vi "Update Timestamp.vi"(6 "Offset (-1 default)":i32=-1, 8 "error in (no error)":errorcluster, 9 "New TAI Time (ns)":i64, 10 "Bytes in":u8[](array[numeric]), 11 "pcap Parse and Build in":refnum<class "pcap_Parse_Build_CIF.lvclass">) -> (0 "error out":errorcluster, 2 "Bytes out":u8[](array[numeric]), 3 "pcap Parse and Build out":refnum<class "pcap_Parse_Build_CIF.lvclass">)   [LabVIEW 2021, in "pcap_Parse_Build_CIF.lvclass"]
doc: "Update the timestamp in-line with the byte array. This is useful for changing time offset of existing data. \n\nIf called after the Parse Packet Header then the offset can be left at the default -1. It will automatically back-up one header set from the current offset. If a value other than -1 is provided it will update the bytes at that location. There is no check to verify location in the byte stream so it is possible to corrupt data if incorrect offsets are used."
uses:
  pcap_Parse_Build_CIF.lvclass
  pcap_Parse_Build_CIF.lvclass/pcap_Parse_Build_CIF.ctl
  Typedef/Errors.ctl
  e9022ed4-8435-466f-84f6-b9a136e00ec6.vi
  b7a2a79d-019e-453d-9ead-29c6d68c4f86.vi
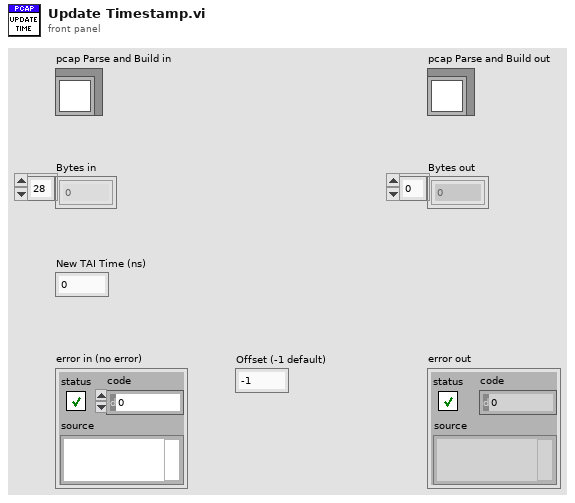
[diagram p1: front panel]
types:
  T1 = typedef "pcap_Parse_Build_CIF.lvclass/Errors.ctl" = enum16{"Invalid Global Header", "Out of Data"}
  T2 = typedef "pcap_Parse_Build_CIF.lvclass/Time Format.ctl" = enum16{"us", "ns"}
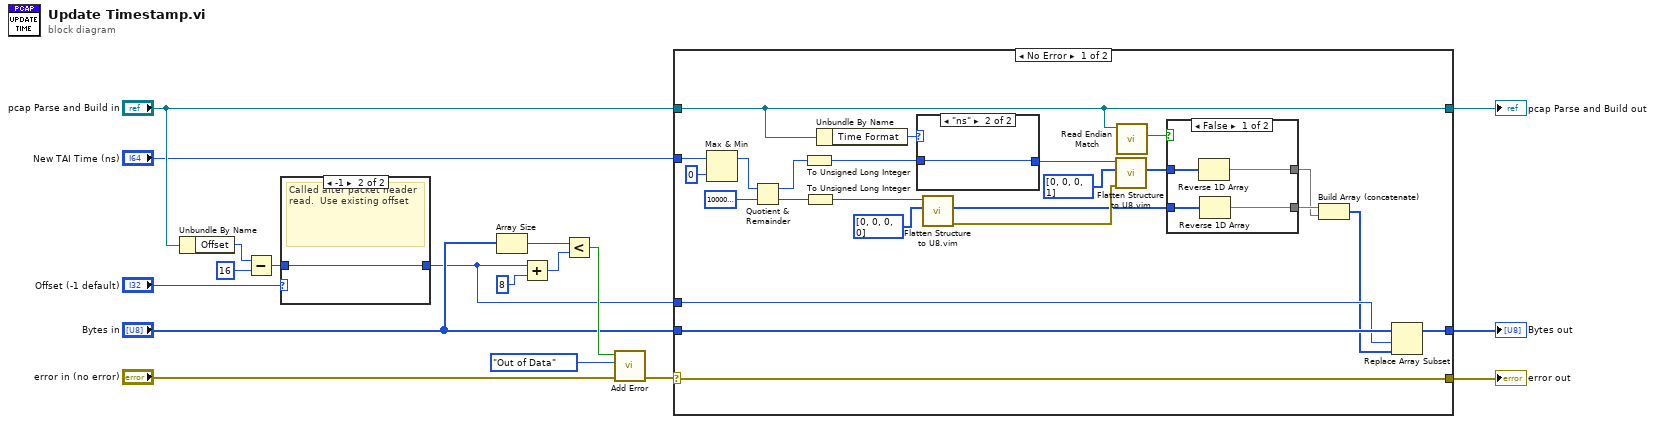
[diagram p0: block diagram]
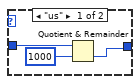
[diagram p4: hidden frame]
diagram:
  n1 = Unbundle By Name("pcap Parse and Build in") -> ("Offset"=w7:i32)
  n2 = Subtract(x=w7, y=16) -> (x-y=w4:i32)
  n3 = case shown="-1" "Offset (-1 default)" {
    selector: "Offset (-1 default)" -> [w18 _]
    tunnel: w4 -> [_ w19]
    tunnel: [w18 w19] -> w3
    frame 0, Default {
      # "Explicit offset provided"
    }
    frame -1 {
      # "Called after packet header read.  Use existing offset"
    }
  }
  n4 = Array Size(array="Bytes in") -> (size(s)=w9:i32)
  n5 = Add(x=w3, y=8 ("length")) -> (x+y=w13:i32)
  n6 = Less?(x=w9, y=w13) -> (x < y?=w11:bool)
  n7 = call "Add Error.vi"("Error"=Errors."Out of Data", "Insert Error"=w11) -> ()  [unwired: 9 in, 1 out]
  n8 = case shown="No Error" "error in (no error)" {
    selector: "error in (no error)" -> [w43 w56]
    tunnel: [w43 w56] -> w16
    tunnel: [w36 w55] -> w14
    tunnel: "pcap Parse and Build in" -> [w36 w55]
    tunnel: "Bytes in" -> [w30 w54]
    tunnel: w3 -> [w29 _]
    tunnel: "New TAI Time (ns)" -> [w37 _]
    tunnel: [w28 w54] -> w1
    frame No Error {
      n9 = Max & Min(x=w37, y=i64 0) -> (max(x,y)=w38:i64)  [unwired: 1 out]
      n10 = Quotient & Remainder(x=w38, y=i64 1000000000) -> (x-y*floor(x/y)=w41:i64, floor(x/y)=w40:i64)
      n11 = To Unsigned Long Integer(number=w41) -> (unsigned 32bit integer=w34:u32)
      n12 = To Unsigned Long Integer(number=w40) -> (unsigned 32bit integer=w33:u32)
      n13 = Unbundle By Name(w36) -> ("Time Format"=w35:T2)
      n14 = case shown="\"ns\"" w35 {
        tunnel: w34 -> [w52 w53]
        tunnel: [w50 w53] -> w31
        frame "us" {
          n15 = Quotient & Remainder(x=w52, y=u32 1000) -> (floor(x/y)=w50:u32)  [unwired: 1 out]
        }
        frame "ns" {
        }
      }
      n16 = call "Flatten Structure to U8.vim"("Flattened Data in"=u8[] [0, 0, 0, 0], "Data to Flatten in"=w33) -> ("error out"=w26:errorcluster, "Flattened Data out"=w22:u8[])  [unwired: 7 in, 1 out]
      n17 = call "Flatten Structure to U8.vim"("error in"=w26, "Flattened Data in"=u8[] [0, 0, 0, 1], "Data to Flatten in"=w31) -> ("Flattened Data out"=w23:u8[])  [unwired: 6 in, 2 out]
      n18 = call "Read Endian Match.vi"("pcap Parse and Build in"=w36) -> ("Endian Match"=w24:bool)  [unwired: 8 in, 2 out]
      n19 = case shown="False" w24 {
        tunnel: w23 -> [w47 w49]
        tunnel: w22 -> [w45 w48]
        tunnel: [w46 w49] -> w20
        tunnel: [w44 w48] -> w21
        frame False {
          n20 = Reverse 1D Array(array=w47) -> (reversed array=w46:u8[])
          n21 = Reverse 1D Array(array=w45) -> (reversed array=w44:u8[])
        }
        frame True {
        }
      }
      n22 = Build Array (concatenate)(w21, w20) -> (w27:u8[])
      n23 = Replace Array Subset(array=w30, new element=w27, index=w29) -> (w28:u8[])
    }
    frame Error {
    }
  }
  "error out" <- w16
  "pcap Parse and Build out" <- w14
  "Bytes out" <- w1
